vi "AI List Refresh.vi"(7 "VarList":refnum<vi>, 8 "错误输入（无错误）":errorcluster, 11 "Device Ref in":T1 format="%.0x") -> (0 "error out":errorcluster, 2 "Channel Refs":T1[](array[typedef]) format="%.0x", 3 "Device Ref out":T1 format="%.0x")   [LabVIEW 2013]
uses:
  <vilib>/K2Labs/HiLab API/Custom Device API/Controls/Custom Device Item Reference.ctl
  <vilib>/K2Labs/HiLab API/Custom Device API/Controls/Custom Device Channel Type.ctl
  MeasurementType.ctl
  AI Terminal Configuration.ctl
  <vilib>/K2Labs/HiLab API/Custom Device API/Configuration/Item Properties/Get Item Property/Get Item Property.xnode
  <vilib>/K2Labs/HiLab API/Custom Device API/Custom Device API Library.lvlib
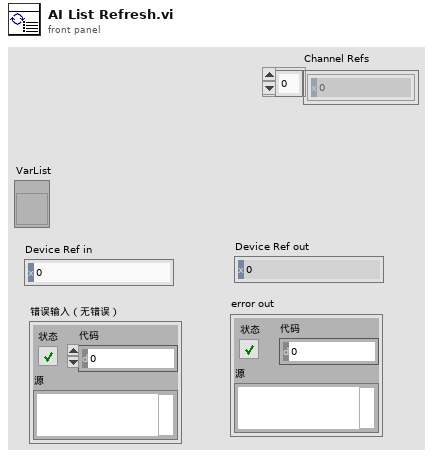
[diagram p1: front panel]
types:
  T1 = typedef "Custom Device API Library.lvlib/Custom Device Item Reference.ctl" = u64
  T2 = typedef "Custom Device API Library.lvlib/Custom Device Channel Type.ctl" = enum16{"Input", "Output"}
  T3 = typedef "AI Terminal Configuration.ctl" = enum16{"默认", "RSE", "NRSE", "差分", "伪差分"}
  T4 = typedef "MeasurementType.ctl" = enum16{"Voltage", "Current", "More:Voltage:Custom with Excitation", "More:Current:Custom with Excitation", "Frequency", "Period", "Resistance", "Temperature:Thermocouple", "Temperature:Thermistor", "Temperature:RTD", "Temperature:Built-in Sensor", "Strain Gage"}
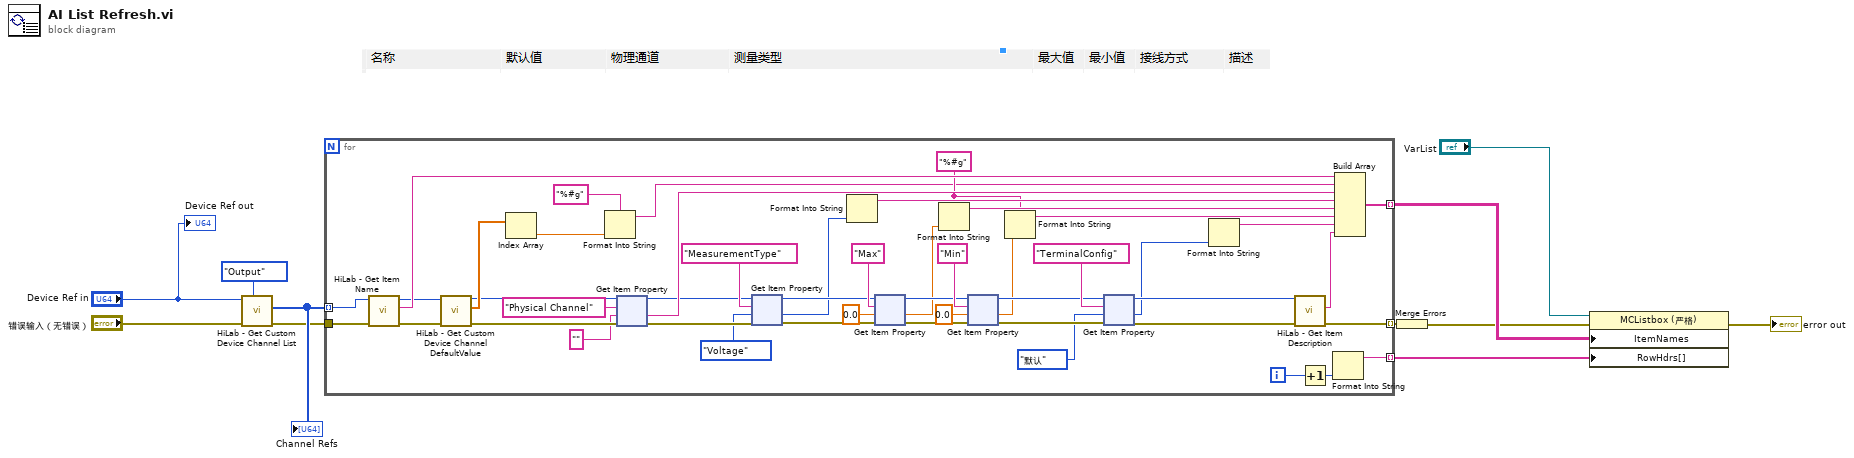
[diagram p0: block diagram]
diagram:
  n1 = call <vilib>:"HiLab - Get Custom Device Channel List.vi"("Type"=Custom_Device_Channel_Type."Output", "error in (no error)"="错误输入（无错误）", "Device Ref in"="Device Ref in") -> ("error out"=w7:errorcluster, "Channel Refs"=w8:T1[])  [unwired: 6 in, 1 out]
  "Channel Refs" <- w8
  n2 = for {
    tunnel: w8 -> [w56] mode=indexing
    tunnel: w7 -> [w57]
    tunnel: [w58] -> w9 mode=indexing
    tunnel: [w46] -> w5 mode=indexing
    tunnel: [w43] -> w2 mode=indexing
    i -> [w44]
    w23 = "%#g" ("格式字符串")
    n3 = call <vilib>:"HiLab - Get Item Name.vi"("error in (no error)"=w57, "Item Ref in"=w56) -> ("error out"=w48:errorcluster, "Name"=w51:string, "Item Ref out"=w49:T1)  [unwired: 6 in, 1 out]
    n4 = call <vilib>:"HiLab - Get Custom Device Channel DefaultValue.vi"("error in (no error)"=w48, "Channel Ref in"=w49) -> ("error out"=w52:errorcluster, "DefaultValue"=w53:dbl[], "Channel Ref out"=w47:T1)  [unwired: 6 in, 1 out]
    n5 = Index Array(array=w53) -> (element=w17:dbl)  [unwired: 1 in]
    n6 = Format Into String(format string="%#g" ("格式字符串"), w17) -> (resulting string=w16:string)  [unwired: 2 in, 1 out]
    n7 = xnode "Get Item Property"("Item Ref in"=w47, "Property Name"="Physical Channel", "Default Value"="", "error in (no error)"=w52) -> ("Item Ref out"=w31:T1, "Value"=w50:string, "error out"=w30:errorcluster)  [unwired: 1 out]
    n8 = xnode "Get Item Property"("Item Ref in"=w31, "Property Name"="MeasurementType", "Default Value"=MeasurementType."Voltage" ("MeasurementType"), "error in (no error)"=w30) -> ("Item Ref out"=w34:T1, "Value"=w28:T4, "error out"=w33:errorcluster)  [unwired: 1 out]
    n9 = Format Into String(w28) -> (resulting string=w27:string)  [unwired: 3 in, 1 out]
    n10 = xnode "Get Item Property"("Item Ref in"=w34, "Property Name"="Max", "Default Value"=0.0, "error in (no error)"=w33) -> ("Item Ref out"=w35:T1, "Value"=w25:dbl, "error out"=w36:errorcluster)  [unwired: 1 out]
    n11 = Format Into String(format string=w23, w25) -> (resulting string=w26:string)  [unwired: 2 in, 1 out]
    n12 = xnode "Get Item Property"("Item Ref in"=w35, "Property Name"="Min", "Default Value"=0.0, "error in (no error)"=w36) -> ("Item Ref out"=w38:T1, "Value"=w24:dbl, "error out"=w37:errorcluster)  [unwired: 1 out]
    n13 = Format Into String(format string=w23, w24) -> (resulting string=w22:string)  [unwired: 2 in, 1 out]
    n14 = xnode "Get Item Property"("Item Ref in"=w38, "Property Name"="TerminalConfig", "Default Value"=AI_Terminal_Configuration."默认" ("Terminal Configuration"), "error in (no error)"=w37) -> ("Item Ref out"=w29:T1, "Value"=w21:T3, "error out"=w32:errorcluster)  [unwired: 1 out]
    n15 = Format Into String(w21) -> (resulting string=w20:string)  [unwired: 3 in, 1 out]
    n16 = call <vilib>:"HiLab - Get Item Description.vi"("error in (no error)"=w32, "Item Ref in"=w29) -> ("error out"=w46:errorcluster, "Discription"=w55:string)  [unwired: 6 in, 2 out]
    n17 = Increment(x=w44) -> (x+1=w45:i32)
    n18 = Format Into String(w45) -> (resulting string=w43:string)  [unwired: 3 in, 1 out]
    n19 = Build Array(w51, w16, w50, w27, w26, w22, w20, w55) -> (w58:string[])
  }
  n20 = Merge Errors(w5) -> (w3:errorcluster)
  n21 = property class="MCListbox (严格)"(reference="VarList", error in=w3, "ItemNames"=w9, "RowHdrs[]"=w2) -> (error out=→"error out":errorcluster)  [unwired: 1 out]
  "Device Ref out" <- "Device Ref in"
